vi "caiquan1.vi"(8 "错误输入（无错误）":errorcluster, 10 "挑战者输入":u16, 11 ".NET引用句柄输入":refnum<k24>) -> (0 "错误输出":errorcluster, 1 "IsEmpty":bool, 2 "挑战者输出":u16, 3 ".NET引用句柄输出":refnum<k24>, 4 "Count":i32)   [LabVIEW 2016]
uses:
  D:/Program Files (x86)/National Instruments/LabVIEW 2016/vi.lib/MakerHub/Leap/Private/Libs/LeapCSharp.NET3.5.dll
  Program Files (x86)/National Instruments/LabVIEW 2016/vi.lib/MakerHub/Leap/Private/Libs/LeapCSharp.NET3.5.dll
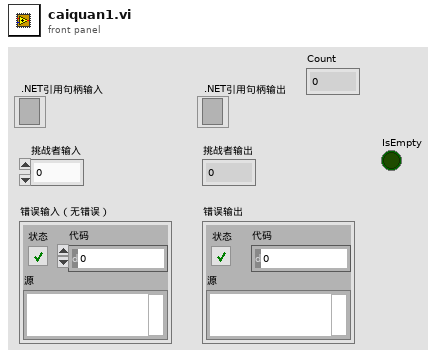
[diagram p1: front panel]
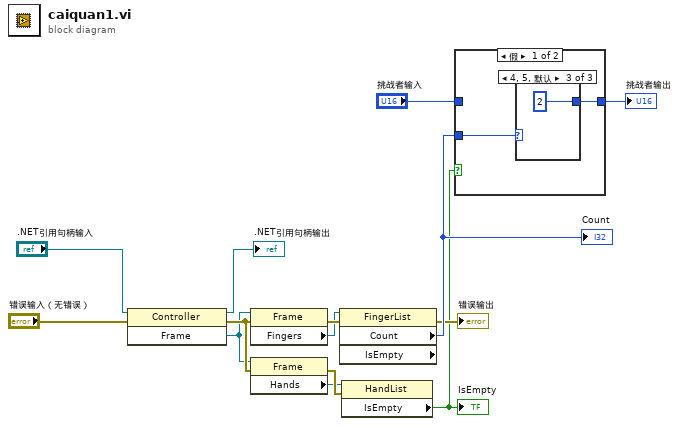
[diagram p0: block diagram]
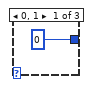
[diagram p2: hidden frame]
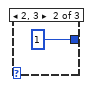
[diagram p3: hidden frame]
diagram:
  n1 = invoke class="Controller" method="Frame"(reference=".NET引用句柄输入", error in="错误输入（无错误）") -> (reference out=→".NET引用句柄输出":refnum<k24>, error out=w8:errorcluster, "Frame"=w7:refnum<k24>)  [unwired: 1 in]
  n2 = property class="Frame"(reference=w7, error in=w8) -> (error out=w11:errorcluster, "Fingers"=w1:refnum<k24>)  [unwired: 1 out]
  n3 = property class="Frame"(reference=w7, error in=w8) -> (error out=w10:errorcluster, "Hands"=w9:refnum<k24>)  [unwired: 1 out]
  n4 = property class="FingerList" props=["Count", "IsEmpty"](reference=w1, error in=w11) -> (error out=→"错误输出":errorcluster, "Count"=w12:i32)  [unwired: 2 out]
  "Count" <- w12
  n5 = property class="HandList"(reference=w9, error in=w10) -> ("IsEmpty"=w2:bool)  [unwired: 2 out]
  "IsEmpty" <- w2
  n6 = case shown="假" w2 {
    tunnel: w12 -> [w16 _]
    tunnel: [w15 w20] -> w14
    tunnel: "挑战者输入" -> [_ w20]
    frame False {
      n7 = case shown="4, 5, 默认" w16 {
        tunnel: [u16 0 ("挑战者") u16 1 ("挑战者") u16 2 ("挑战者")] -> w15
        frame 0, 1 {
        }
        frame 2, 3 {
        }
        frame 4, 5, Default {
        }
      }
    }
    frame True {
    }
  }
  "挑战者输出" <- w14
